vi "calculator.vi"() -> ()   [LabVIEW 2009]
panel:
  in  "stop":bool
  out "Result":dbl
  in  "Ring":u16(ring) items=["addition", "substraction", "multiplication", "division", "reminder"]
  in  "Input 2":dbl
  in  "Input 1":dbl
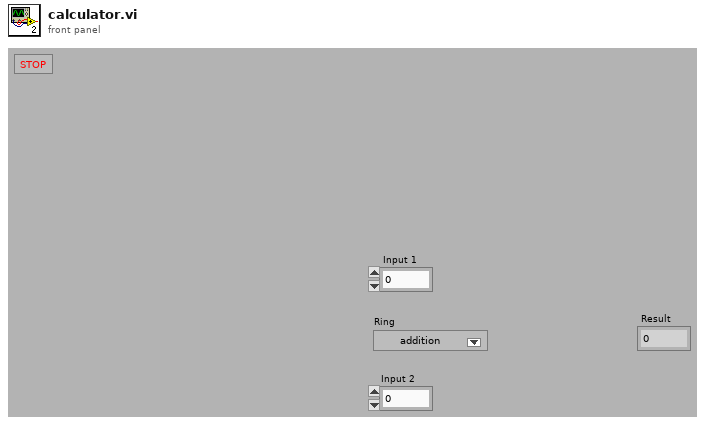
[diagram p1: front panel]
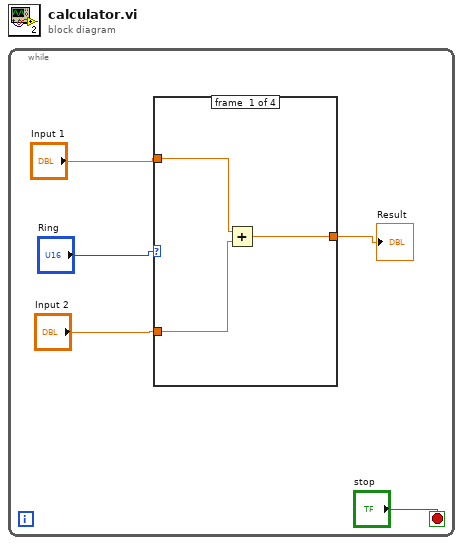
[diagram p0: block diagram]
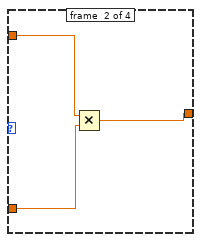
[diagram p2: hidden frame]
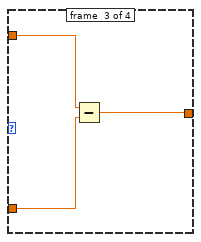
[diagram p3: hidden frame]
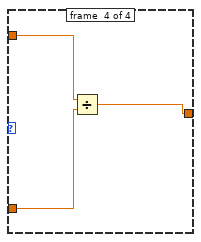
[diagram p4: hidden frame]
diagram:
  n1 = while {
    stop <- "stop" stop-if-true
    n2 = case shown="0, Default" "Ring" {
      tunnel: "Input 1" -> [w8 w11 w14 w17]
      tunnel: "Input 2" -> [w7 w10 w13 w16]
      tunnel: [w6 w9 w12 w15] -> w2
      frame #0 {
        n3 = Add(x=w8, y=w7) -> (x+y=w6:dbl)
      }
      frame #1 {
        n4 = Multiply(x=w11, y=w10) -> (x*y=w9:dbl)
      }
      frame #2 {
        n5 = Subtract(x=w14, y=w13) -> (x-y=w12:dbl)
      }
      frame #3 {
        n6 = Divide(x=w17, y=w16) -> (x/y=w15:dbl)
      }
    }
    "Result" <- w2
  }
